vi "Initialise.vi"(8 "error in (no error)":errorcluster, 10 "Timeout":u32=2000, 11 "Driver in":refnum<class "Driver.lvclass">) -> (0 "error out":errorcluster, 3 "Driver out":refnum<class "Driver.lvclass">)   [LabVIEW 2023, in "HAF.lvlib" / "Driver.lvclass"]
doc: "Configures the Driver to be ready to send Commands to the Instrument."
uses:
  Driver.lvclass
  Driver.lvclass/Driver.ctl
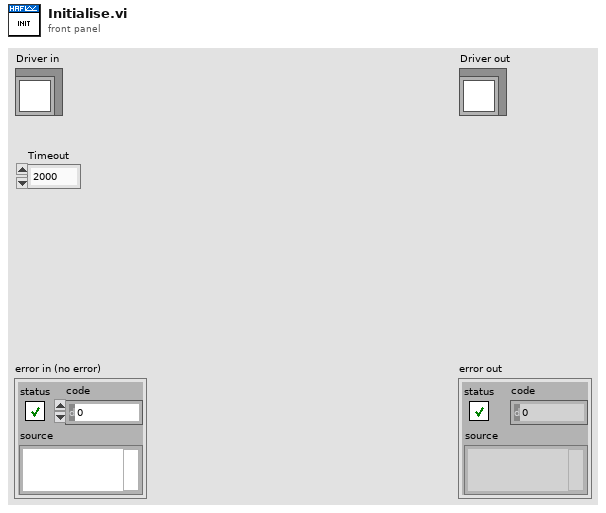
[diagram p1: front panel]
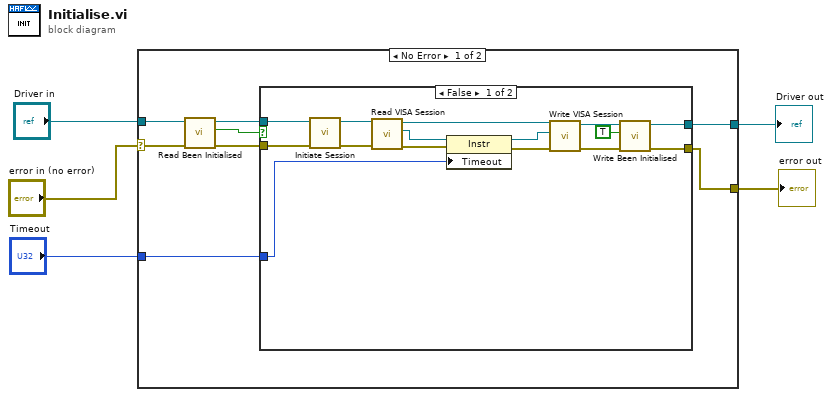
[diagram p0: block diagram]
diagram:
  n1 = case shown="No Error" "error in (no error)" {
    selector: "error in (no error)" -> [w12 w32]
    tunnel: [w6 w32] -> w4
    tunnel: [w7 w31] -> w2
    tunnel: "Driver in" -> [w13 w31]
    tunnel: "Timeout" -> [w8 _]
    frame No Error {
      n2 = call-dynamic "Read Been Initialised.vi"("error in (no error)"=w12, "Driver in"=w13) -> ("error out"=w9:errorcluster, "Been Initialised"=w10:bool, "Driver out"=w11:refnum<class "Driver.lvclass">)  [unwired: 7 in]
      n3 = case shown="False" w10 {
        tunnel: w11 -> [w28 w30]
        tunnel: w9 -> [w27 w29]
        tunnel: w8 -> [w23 _]
        tunnel: [w15 w30] -> w7
        tunnel: [w14 w29] -> w6
        frame False {
          n4 = call-dynamic "Initiate Session.vi"("error in (no error)"=w27, "Driver in"=w28) -> ("error out"=w25:errorcluster, "Driver out"=w26:refnum<class "Driver.lvclass">)  [unwired: 8 in]
          n5 = call-dynamic "Read VISA Session.vi"("error in (no error)"=w25, "Driver in"=w26) -> ("error out"=w22:errorcluster, "VISA Session"=w24:refnum<visa-resource-name>, "Driver out"=w21:refnum<class "Driver.lvclass">)  [unwired: 7 in]
          n6 = property class="Instr"(reference=w24, error in=w22, "Timeout"=w23) -> (reference out=w20:refnum<visa-resource-name>, error out=w19:errorcluster)
          n7 = call-dynamic "Write VISA Session.vi"("error in (no error)"=w19, "VISA Session"=w20, "Driver in"=w21) -> ("error out"=w17:errorcluster, "Driver out"=w18:refnum<class "Driver.lvclass">)  [unwired: 7 in]
          n8 = call-dynamic "Write Been Initialised.vi"("error in (no error)"=w17, "Been Initialised"=TRUE, "Driver in"=w18) -> ("error out"=w14:errorcluster, "Driver out"=w15:refnum<class "Driver.lvclass">)  [unwired: 7 in]
        }
        frame True {
          # "Already initialised, do nothing"
        }
      }
    }
    frame Error {
    }
  }
  "error out" <- w4
  "Driver out" <- w2
